vi "util.file.record.vi"(6 "Operation(Read)":enum16{"Read File", "Write File"}(ring), 8 "error in":errorcluster, 9 "clk":dbl=-1.0, 10 "value":dbl, 11 "path.* in":string="folder1\\folder2\\filename.log") -> (0 "error out":errorcluster, 1 "Last Record out":dbl[](array[numeric]), 2 "cluster":cluster{"X":dbl[], "Y":dbl[]}, 3 "Selected Folder":path=path "C:/interface/log/folder1/folder2/2024_07_03__filename.log")   [LabVIEW 2024]
doc: "Illustrates the various data types that the XY Graph accepts. Use the XY Graph to display data that is not uniformly distributed along the X-axis. This is particularly useful when displaying data that was sampled at a variable rate. The XY Graph is also useful for displaying data that is formatted as (X,Y) pairs."
uses:
  controls/typePathSelector.ctl
  <vilib>/Utility/error.llb/Clear Errors.vi
  <vilib>/Utility/file.llb/Write Delimited Spreadsheet (string).vi
  <vilib>/Utility/file.llb/Read Delimited Spreadsheet (DBL).vi
panel:
  out "Multiple Plots (X Array and Y Array)":cluster{"all rows":dbl[], "all rows":dbl[]}(graph)
  # "example:\nfolder1\\folder2\\filename.*"
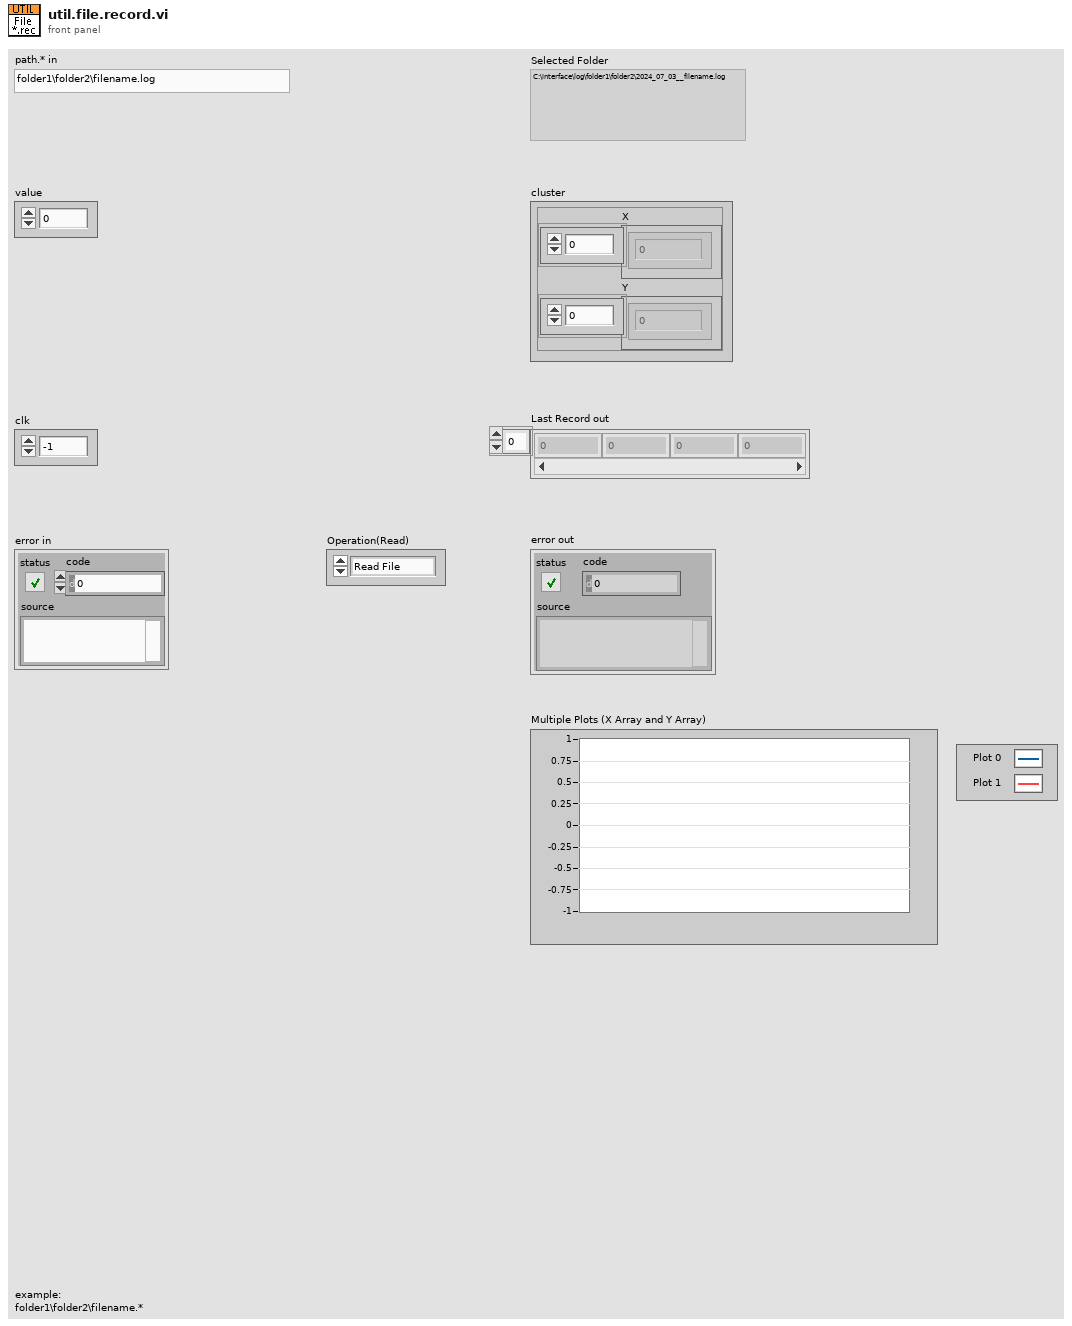
[diagram p1: front panel]
types:
  T1 = typedef "typePathSelector.ctl" = enum16{"DIR_PROCS", "DIR_CONFIG", "DIR_TEMPLATE", "DIR_IO_FILE", "DIR_RECORD", "DIR_LOG", "DIR_RUNTIME", "DIR_PRESET", "DIR_INI"}
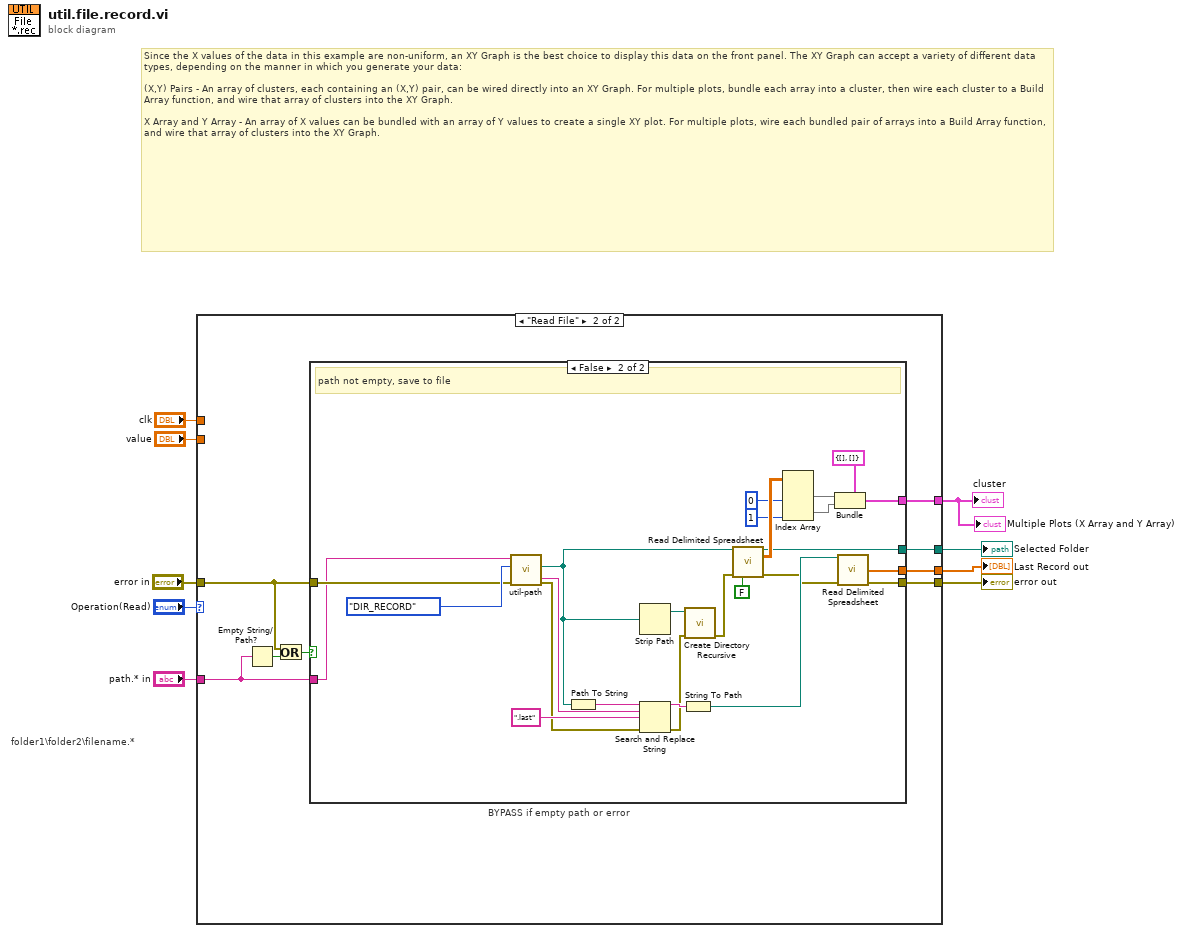
[diagram p0: block diagram]
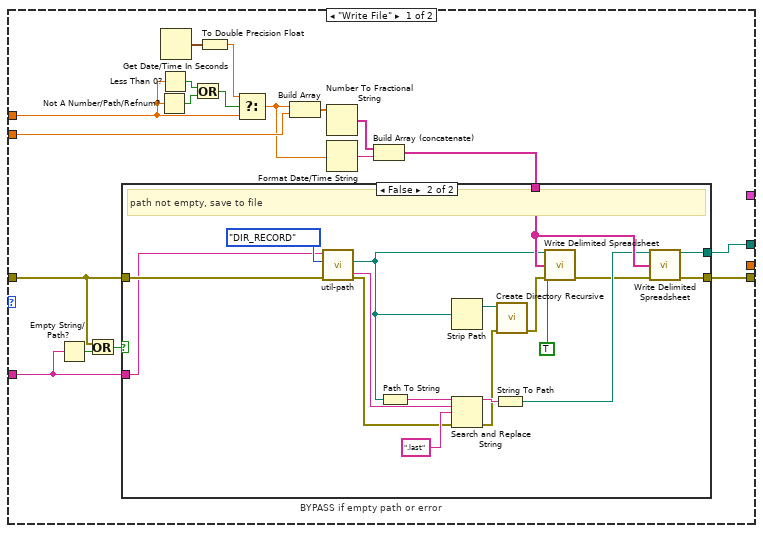
[diagram p2: hidden frame]
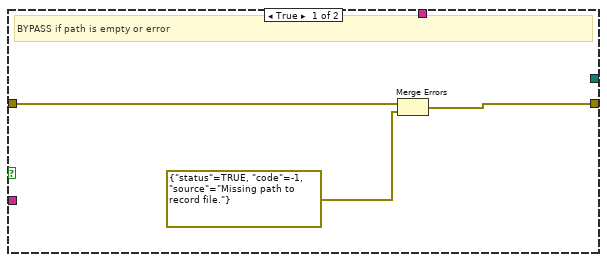
[diagram p3: hidden frame]
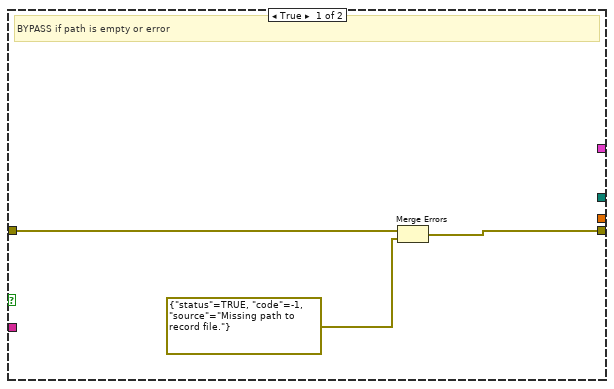
[diagram p4: hidden frame]
diagram:
  # "folder1\\folder2\\filename.*"
  # "Since the X values of the data in this example are non-uniform, an XY Graph is the best choice to display this data on the front panel. The XY Graph can accept a variety of different data types, depending on the manner in which you generate your data:\n\n(X,Y) Pairs - An array of clusters, each containing an (X,Y) pair, can be wired directly into an XY Graph. For multiple plots, bundle each array into a cluster, then wire each cluster to a Build Array function, and wire that array of clusters into the XY Graph.\n\nX Array and Y Array - An array of X values can be bundled with an array of Y values to create a single XY plot. For multiple plots, wire each bundled pair of arrays into a Build Array function, and wire that array of clusters into the XY Graph."
  n1 = case shown="\"Read File\"" "Operation(Read)" {
    tunnel: "value" -> [w27 _]
    tunnel: "clk" -> [w26 _]
    tunnel: [w24 w56] -> w7
    tunnel: [w23 w55] -> w6
    tunnel: "error in" -> [w22 w54]
    tunnel: "path.* in" -> [w21 w53]
    tunnel: [_ w50] -> w2
    tunnel: [_ w49] -> w1
    frame "Write File" {
      n2 = Empty String/Path?(string/path=w21) -> (empty?=w11:bool)
      n3 = Or(x=w22, y=w11) -> (x .or. y?=w10:bool)
      n4 = Not A Number/Path/Refnum?(number/path/refnum=w26) -> (NaN/Path/Refnum?=w19:bool)
      n5 = Less Than 0?(x=w26) -> (x < 0?=w17:bool)
      n6 = Get Date/Time In Seconds() -> (seconds since 1Jan1904=w20:timestamp)
      n7 = Or(x=w17, y=w19) -> (x .or. y?=w18:bool)
      n8 = To Double Precision Float(number=w20) -> (double precision float=w13:dbl)
      n9 = Select(t=w13, s=w18, f=w26) -> (s? t:f=w12:dbl)
      n10 = Build Array(w12, w27) -> (w16:dbl[])
      n11 = Number To Fractional String(number=w16) -> (F-format string=w14:string[])  [unwired: 3 in]
      n12 = Format Date/Time String(seconds (now)=w12) -> (date/time string=w15:string)  [unwired: 2 in]
      n13 = Build Array (concatenate)(w14, w15) -> (w25:string[])
      n14 = case "BYPASS if empty path or error" shown="False" w10 {
        tunnel: w25 -> [_ w40]
        tunnel: [w29 w41] -> w24
        tunnel: [_ w42] -> w23
        tunnel: w22 -> [w30 w45]
        tunnel: w21 -> [_ w44]
        frame True {
          # "BYPASS if path is empty or error"
          n15 = Merge Errors(w30, errorcluster {"status"=TRUE, "code"=-1, "source"="Missing path to record file."} ("error in")) -> (w29:errorcluster)
        }
        frame False {
          # "path not empty, save to file"
          n16 = call "util-path.vi"("error in"=w45, "Selected Folder (PROCS)"=typePathSelector."DIR_RECORD" ("*Folder Select"), "append path (ie. folder\\filename.*)"=w44) -> ("error out"=w34:errorcluster, "SelectedPath"=w39:path, ".extension (.prc)"=w37:string)  [unwired: 4 in, 2 out]
          n17 = Path To String(path=w39) -> (string=w38:string)
          n18 = Strip Path(path=w39) -> (stripped path=w43:path)  [unwired: 1 out]
          n19 = Search and Replace String(input string=w38, search string=w37, replace string=".last" ("replace string (\"\")"), error in=w34) -> (result string=w35:string, error out=w32:errorcluster)  [unwired: 4 in, 2 out]
          n20 = String To Path(string=w35) -> (path=w33:path)
          n21 = call <vilib>:"Create Directory Recursive.vi"("error in (no error)"=w32, "directory"=w43) -> ("error out"=w46:errorcluster)  [unwired: 3 in, 2 out]
          n22 = call-poly <vilib>:"Write Delimited Spreadsheet.vi"("file path (dialog if empty)"=w39, "1D data"=w40, "append to file? (new file:F)"=TRUE, "error in (no error)"=w46) -> ("error out"=w31:errorcluster)  [unwired: 10 in, 1 out]
          n23 = call-poly <vilib>:"Write Delimited Spreadsheet.vi"("file path (dialog if empty)"=w33, "1D data"=w40, "error in (no error)"=w31) -> ("new file path (Not A Path if cancelled)"=w42:path, "error out"=w41:errorcluster)  [unwired: 11 in]
        }
      }
    }
    frame "Read File" {
      n24 = Empty String/Path?(string/path=w53) -> (empty?=w52:bool)
      n25 = Or(x=w54, y=w52) -> (x .or. y?=w51:bool)
      n26 = case "BYPASS if empty path or error" shown="False" w51 {
        tunnel: [w58 w78] -> w56
        tunnel: [_ w61] -> w55
        tunnel: w54 -> [w59 w81]
        tunnel: w53 -> [_ w80]
        tunnel: [_ w68] -> w50
        tunnel: [_ w62] -> w49
        frame True {
          # "BYPASS if path is empty or error"
          n27 = Merge Errors(w59, errorcluster {"status"=TRUE, "code"=-1, "source"="Missing path to record file."} ("error in")) -> (w58:errorcluster)
        }
        frame False {
          # "path not empty, save to file"
          n28 = call "util-path.vi"("error in"=w81, "Selected Folder (PROCS)"=typePathSelector."DIR_RECORD" ("*Folder Select"), "append path (ie. folder\\filename.*)"=w80) -> ("error out"=w72:errorcluster, "SelectedPath"=w77:path, ".extension (.prc)"=w75:string)  [unwired: 4 in, 2 out]
          n29 = Path To String(path=w77) -> (string=w76:string)
          n30 = Strip Path(path=w77) -> (stripped path=w79:path)  [unwired: 1 out]
          n31 = Search and Replace String(input string=w76, search string=w75, replace string=".last" ("replace string (\"\")"), error in=w72) -> (result string=w73:string, error out=w70:errorcluster)  [unwired: 4 in, 2 out]
          n32 = String To Path(string=w73) -> (path=w71:path)
          n33 = call <vilib>:"Create Directory Recursive.vi"("error in (no error)"=w70, "directory"=w79) -> ("error out"=w82:errorcluster)  [unwired: 3 in, 2 out]
          n34 = call-poly <vilib>:"Read Delimited Spreadsheet.vi"("file path (dialog if empty)"=w77, "error in (no error)"=w82, "transpose? (F)"=FALSE ("append to file? (new file:F)")) -> ("new file path (Not A Path if cancelled)"=w61:path, "all rows"=w65:dbl[][], "error out"=w69:errorcluster)  [unwired: 7 in, 3 out]
          n35 = Index Array(array=w65, index (col) #1=0 ("disabled index (col)"), index (col) #2=1 ("index (col)")) -> (element #1=w67:dbl[], element #2=w66:dbl[])  [unwired: 2 in]
          n36 = Bundle(cluster=cluster{"X":dbl[], "Y":dbl[]} {"X"=[], "Y"=[]}, "X"=w67, "Y"=w66) -> (w62:cluster{"X":dbl[], "Y":dbl[]})
          n37 = call-poly <vilib>:"Read Delimited Spreadsheet.vi"("file path (dialog if empty)"=w71, "error in (no error)"=w69) -> ("first row"=w68:dbl[], "error out"=w78:errorcluster)  [unwired: 8 in, 4 out]
        }
      }
    }
  }
  "error out" <- w7
  "Selected Folder" <- w6
  "Last Record out" <- w2
  "Multiple Plots (X Array and Y Array)" <- w1
  "cluster" <- w1
